vi "test_Command and Response with Byte count wait time.vi"(8 "error in (no error)":errorcluster, 11 "TestCase in":refnum<class "Instrument Addon Host API Tests.lvclass">) -> (0 "error out":errorcluster, 3 "TestCase out":refnum<class "Instrument Addon Host API Tests.lvclass">)   [LabVIEW 2018, in "Instrument Addon Host API Tests.lvclass"]
uses:
  Instrument Addon Host API Tests.lvclass
  Addon/Addon Shared/Types/Buffered RT Instrument Command.ctl
  Addon/Addon Shared/Types/Response Wait Type.ctl
  <vilib>/addons/_JKI Toolkits/VI Tester/TestCase.llb/TestCase.lvclass
  APIs/Host Automation API/Instrument Host Automation API.lvlib
  Addon/Addon Shared/Instrument Addon Shared.lvlib
  C:/Program Files (x86)/National Instruments/LabVIEW 2018/vi.lib/addons/_JKI Toolkits/VI Tester/TestCase.llb/TestCase.lvclass
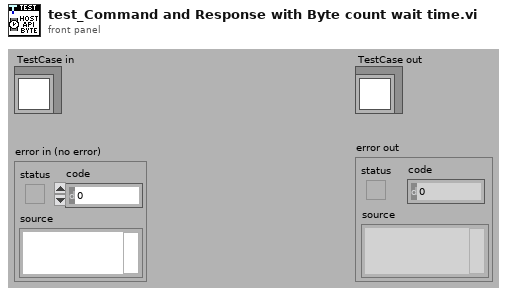
[diagram p1: front panel]
types:
  T1 = typedef "Instrument Addon Shared.lvlib/Buffered RT Instrument Command.ctl" = cluster{"Command":string, "Response Expected?":bool, "Wait Type":T2, "Wait Value":dbl}
  T2 = typedef "Instrument Addon Shared.lvlib/Response Wait Type.ctl" = enum16{"Byte Count", "Wait sec"}
  T3 = typedef "NI STM.lvlib/TCP Connection Info.ctl" = cluster{"connection ID":refnum<k5>, "meta data":T4[]}
  T4 = typedef "NI STM.lvlib/MetaDataElement.ctl" = string
  T5 = typedef "Instrument Addon Shared.lvlib/Buffered RT Instrument Request.ctl" = cluster{"Response":string, "Error":errorcluster}
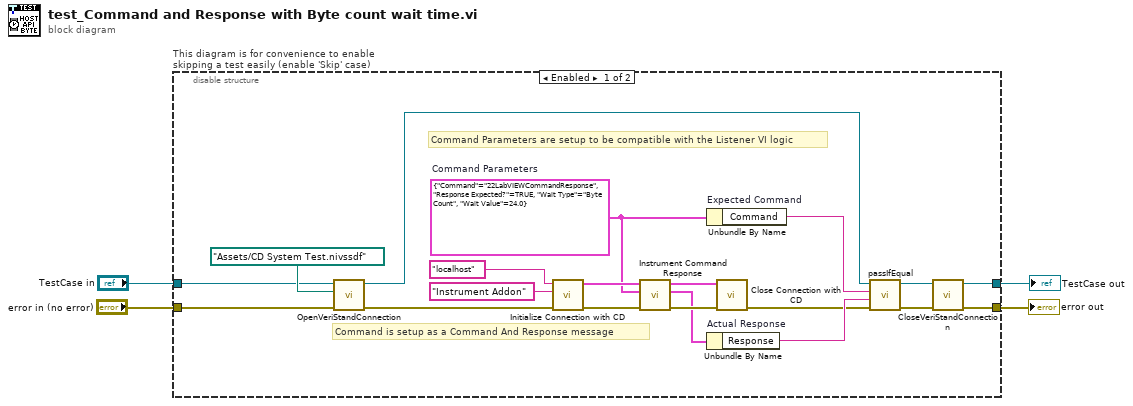
[diagram p0: block diagram]
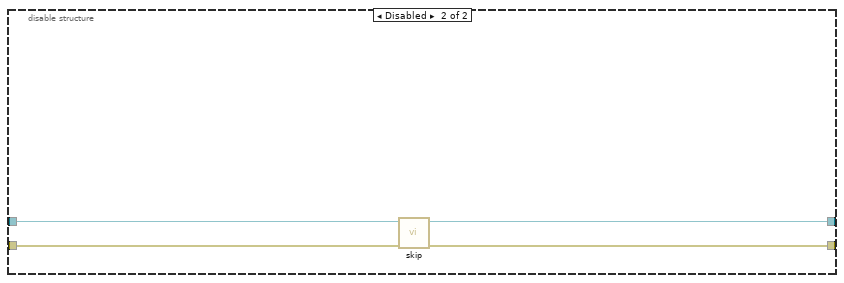
[diagram p2: hidden frame]
diagram:
  n1 = disable-structure "This diagram is for convenience to enable skipping a test easily (enable 'Skip' case)" shown="Enabled" {
    disable-tunnel: "TestCase in" -> [w22 w28]
    disable-tunnel: [w20 w26] -> w1
    disable-tunnel: [w21 w27] -> w3
    disable-tunnel: "error in (no error)" -> [w23 w25]
    frame Enabled {
      w5 = T1 {"Command"="22LabVIEWCommandResponse", "Response Expected?"=TRUE, "Wait Type"=enum."Byte Count", "Wait Value"=24.0}  # Command Parameters
      # "Command Parameters are setup to be compatible with the Listener VI logic"
      # "Command is setup as a Command And Response message"
      n2 = call-dynamic "OpenVeriStandConnection.vi"("error in (no error)"=w23, "System Definition File"=path "Assets/CD System Test.nivssdf", "VeriStand Test Case in"=w22) -> ("error out"=w6:errorcluster, "VeriStand Test Case out"=w18:refnum<class "Instrument Addon Host API Tests.lvclass">)  [unwired: 6 in, 1 out]
      n3 = call "Initialize Connection with CD.vi"("error in (no error)"=w6, "TCP Service"="Instrument Addon", "IP Address"="localhost") -> ("error out"=w11:errorcluster, "connection info out"=w10:T3)  [unwired: 7 in]
      n4 = call "Instrument Command Response.vi"("error in (no error)"=w11, "Command Parameters"=w5, "Comm.Info"=w10) -> ("error out"=w9:errorcluster, "Response"=w7:T5, "Comm.Info"=w8:T3)  [unwired: 5 in, 1 out]
      n5 = Unbundle By Name "Expected Command"(w5) -> ("Command"=w15:string)
      n6 = Unbundle By Name "Actual Response"(w7) -> ("Response"=w16:string)
      n7 = call "Close Connection with CD.vi"("error in"=w9, "Comm.Info"=w8) -> ("error out"=w14:errorcluster)  [unwired: 9 in]
      n8 = call-dynamic "passIfEqual.vi"("error in (no error)"=w14, "y"=w16, "x"=w15, "TestCase in"=w18) -> ("error out"=w19:errorcluster, "TestCase out"=w17:refnum<class "Instrument Addon Host API Tests.lvclass">)  [unwired: 6 in]
      n9 = call-dynamic "CloseVeriStandConnection.vi"("error in (no error)"=w19, "VeriStand Test Case in"=w17) -> ("error out"=w21:errorcluster, "VeriStand Test Case out"=w20:refnum<class "Instrument Addon Host API Tests.lvclass">)  [unwired: 8 in]
    }
    frame Disabled {
      # "skip test result while test is under development"
      n10 = call <vilib>:"skip.vi"("error in (no error)"=w25, "TestCase in"=w28) -> ("error out"=w27:errorcluster, "TestCase out"=w26:refnum<class "Instrument Addon Host API Tests.lvclass">)  [unwired: 8 in]
    }
  }
  "error out" <- w3
  "TestCase out" <- w1
